vi "Prompt Convert 1.8 to 1.9.vi"(0 "Prompt 1.8 Test Parameters":T3) -> (1 "Datasheets":T1, 2 "Prompt 1.9 Test Parameters":T2)   [LabVIEW 2011]
uses:
  TypeDefs/Prompt Test Parameters v1.8.ctl
  TypeDefs/Prompt Test Parameters.ctl
  Test Datasheets v1.0-4.0.ctl
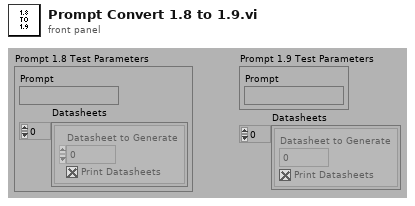
[diagram p1: front panel]
types:
  T1 = typedef "Test Datasheets v1.0-4.0.ctl" = cluster{"Datasheet to Generate":i32, "Print Datasheets":bool}[]
  T2 = typedef "Prompt Test Parameters.ctl" = cluster{"Prompt":string}
  T3 = typedef "Prompt Test Parameters v1.8.ctl" = cluster{"Prompt":string, "Datasheets":cluster{"Datasheet to Generate":i32, "Print Datasheets":bool}[]}
  T4 = cluster{"Datasheet to Generate":i32, "Print Datasheets":bool}[]
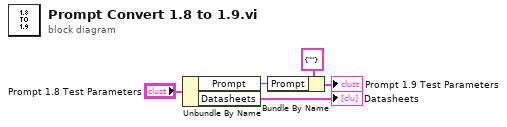
[diagram p0: block diagram]
diagram:
  n1 = Unbundle By Name("Prompt 1.8 Test Parameters") -> ("Prompt"=w4:string, "Datasheets"=→"Datasheets":T4)
  n2 = Bundle By Name(cluster=T2 {"Prompt"=""} ("Prompt Test Parameters"), "Prompt"=w4) -> (→"Prompt 1.9 Test Parameters":T2)
